vi "AI_Joystick_Manual.vi"() -> ()   [LabVIEW 2016]
uses:
  <vilib>/myRIO/Instrument Drivers/Onboard IO/AI/typedefs/AI Reference.ctl
  <vilib>/myRIO/Common/Instrument Driver Framework/Utilities/typedefs/myRIO Generic Hardware Reference.ctl
  <vilib>/myRIO/Common/Instrument Driver Framework/Utilities/typedefs/Hardware Version Enum.ctl
  <vilib>/myRIO/Common/Instrument Driver Framework/Utilities/typedefs/myRIO v1.0 Reference.ctl
  <vilib>/myRIO/Common/Instrument Driver Framework/Utilities/typedefs/Generic FPGA Reference.ctl
  <vilib>/myRIO/Common/Instrument Driver Framework/myRIO v1.0/AI/typedefs/AI Channels List.ctl
  <vilib>/myRIO/Common/Instrument Driver Framework/myRIO v1.0/AI/typedefs/AI Channels Enum.ctl
  <vilib>/myRIO/Common/Instrument Driver Framework/Utilities/typedefs/Analog Scaling Constants List.ctl
  <vilib>/myRIO/Common/Instrument Driver Framework/Utilities/typedefs/Analog Scaling Constants.ctl
  <vilib>/userdefined/High Color/nirio_resource_hc.ctl
  <vilib>/myRIO/Common/Instrument Driver Framework/Utilities/vis/Is FPGA Ref Available.vi
  <vilib>/myRIO/Common/Instrument Driver Framework/myRIO v1.0/AI/vis/myRIO v1.1 Open AI.vi
  <vilib>/myRIO/Instrument Drivers/Onboard IO/AI/vis/Read.vi
  <vilib>/myRIO/Common/Instrument Driver Framework/Utilities/vis/Validate Channels.vi
  <vilib>/myRIO/Common/Instrument Driver Framework/myRIO v1.0/AI/vis/myRIO v1.0 Reserve AI.vi
  <vilib>/myRIO/Common/Instrument Driver Framework/myRIO v1.0/AI/vis/myRIO v1.0 Build MUX Configuration AI.vi
  <vilib>/myRIO/Common/Instrument Driver Framework/myRIO v1.0/Resource Manager/vis/myRIO v1.0 Reserve Channel List.vi
  <vilib>/myRIO/Common/Instrument Driver Framework/myRIO v1.0/Resource Manager/vis/myRIO v1.0 Reserve Channel.vi
  <vilib>/myRIO/Common/Instrument Driver Framework/myRIO v1.0/Resource Manager/vis/myRIO v1.0 Unreserve Channel.vi
  <vilib>/myRIO/Common/Instrument Driver Framework/myRIO v1.0/Resource Manager/vis/myRIO v1.0 Build Mutex Name.vi
  <vilib>/Utility/VariantDataType/GetNumericInfo.vi
  <vilib>/Utility/error.llb/Error Cluster From Error Code.vi
  <vilib>/myRIO/Common/Instrument Driver Framework/myRIO v1.0/myRIO v1.1 Open.vi
  <vilib>/myRIO/Common/Instrument Driver Framework/myRIO v1.0/AI/vis/myRIO v1.0 Get Scaling Constants AI.vi
  <vilib>/myRIO/Common/Instrument Driver Framework/Utilities/vis/IO Manager.vi
  <vilib>/myRIO/Common/Instrument Driver Framework/Utilities/vis/Configuration Manager.vi
  <vilib>/myRIO/Common/Instrument Driver Framework/myRIO v1.0/myRIO v1.0 Close.vi
  <vilib>/myRIO/Common/Instrument Driver Framework/myRIO v1.0/AI/vis/myRIO v1.0 Read AI.vi
  <vilib>/myRIO/Express VI/Onboard IO/AI/AI Express VI.xnode
  <vilib>/myRIO/Instrument Drivers/Onboard IO/AI/vis/myRIO AI Open.xnode
  <vilib>/myRIO/Instrument Drivers/Onboard IO/AI/AI.lvlib
panel:
  in  "X":dbl=2.0
  in  "y":dbl=2.0
  out "Right Speed":dbl format="%#.1f"
  in  "stop":bool
  out "Reset Encoder":bool
  out "Left Speed":dbl format="%#.1f"
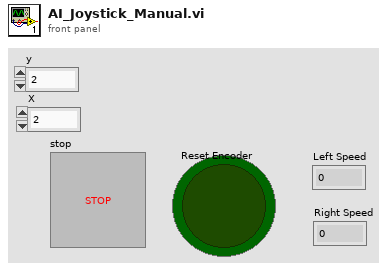
[diagram p1: front panel]
types:
  T1 = typedef "AI.lvlib/AI Reference.ctl" = cluster{"myRIO Reference":T2, "AI Channels List":T6, "AI Scaling Constants List":T8}
  T2 = typedef "myRIO Generic Hardware Reference.ctl" = cluster{"myRIO Model":T3, "myRIO Hardware Reference":T4}
  T3 = typedef "Hardware Version Enum.ctl" = enum16{"Unknown", "myRIO-1900", "myRIO-1950", "roboRIO", "NI ELVIS RIO CM"}
  T4 = typedef "myRIO v1.0 Reference.ctl" = cluster{"Generic FPGA Reference":T5, "Allow multiple opens":bool}
  T5 = typedef "Generic FPGA Reference.ctl" = refnum<k20>
  T6 = typedef "AI Channels List.ctl" = T7[]
  T7 = typedef "AI Channels Enum.ctl" = enum16{"Not Connected", "AudioIn/Left", "AudioIn/Right", "C/AI0", "C/AI1", "A/AI0", "A/AI1", "A/AI2", "A/AI3", "B/AI0", "B/AI1", "B/AI2", "B/AI3", "AI/AI0", "AI/AI1", "AI/AI2", "AI/AI3"}
  T8 = typedef "Analog Scaling Constants List.ctl" = T9[]
  T9 = typedef "Analog Scaling Constants.ctl" = cluster{"LSB Weight (Volts)":dbl, "Offset (Volts)":dbl, "Signed?":bool}
  T10 = typedef "nirio_resource_hc.ctl" = tag
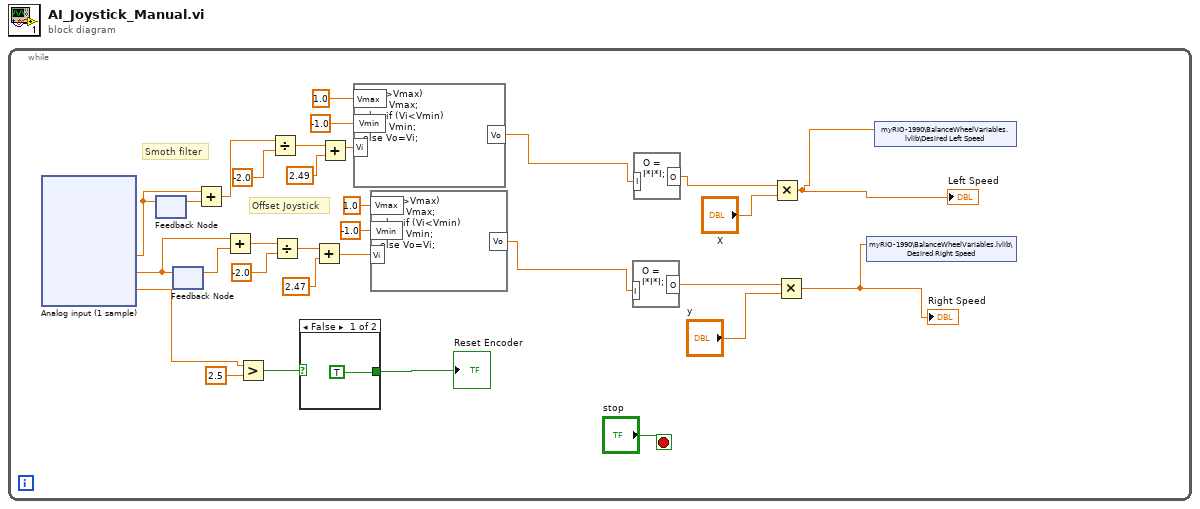
[diagram p0: block diagram]
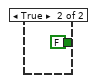
[diagram p2: hidden frame]
diagram:
  n1 = while {
    stop <- "stop" stop-if-true
    # "Offset Joystick"
    # "Smoth filter"
    n2 = xnode "Analog input (1 sample)"() -> ("B/AI2 (Pin 7)"=w18:dbl, "B/AI1 (Pin 5)"=w20:dbl, "B/AI0 (Pin 3)"=w17:dbl)  [unwired: 1 in, 1 out]
    n3 = feedback #1() -> (w27:dbl)  [unwired: 1 in]
    n4 = feedback-in #1(w18) -> ()
    n5 = feedback #2() -> (w23:dbl)  [unwired: 1 in]
    n6 = feedback-in #2(w20) -> ()
    n7 = Add(x=w18, y=w27) -> (x+y=w26:dbl)
    n8 = Add(x=w20, y=w23) -> (x+y=w22:dbl)
    n9 = Greater?(x=w17, y=2.5) -> (0:w30:bool)
    n10 = Divide(x=w26, y=-2.0) -> (x/y=w24:dbl)
    n11 = Divide(x=w22, y=-2.0) -> (x/y=w19:dbl)
    n12 = case shown="False" w30 {
      tunnel: [TRUE ("Boolean 2") FALSE ("Boolean 2")] -> w15
      frame False {
      }
      frame True {
      }
    }
    "Reset Encoder" <- w15
    n13 = Add(x=w19, y=2.47) -> (x+y=w11:dbl)
    n14 = Add(x=w24, y=2.49) -> (x+y=w14:dbl)
    n15 = formula code="if (Vi>Vmax)\nVo = Vmax;\nelse if (Vi<Vmin)\nVo = Vmin;\nelse Vo=Vi;"("Vi"=w14, "Vmin"=-1.0 ("input variable"), "Vmax"=1.0 ("input variable")) -> ("Vo"=w6:dbl)
    n16 = formula code="if (Vi>Vmax)\nVo = Vmax;\nelse if (Vi<Vmin)\nVo = Vmin;\nelse Vo=Vi;"("Vi"=w11, "Vmin"=-1.0 ("input variable"), "Vmax"=1.0 ("input variable")) -> ("Vo"=w4:dbl)
    n17 = formula code="O = I*I*I;"("I"=w4) -> ("O"=w3:dbl)
    n18 = formula code="O = I*I*I;"("I"=w6) -> ("O"=w5:dbl)
    n19 = Multiply(x=w5, y="X") -> (x*y=w2:dbl)
    "Left Speed" <- w2
    n20 = Multiply(x=w3, y="y") -> (x*y=w1:dbl)
    "Right Speed" <- w1
    n21 = shared-variable "myRIO-1990\\BalanceWheelVariables.lvlib\\Desired Right Speed"(w1) -> ()  [unwired: 1 in, 1 out]
    n22 = shared-variable "myRIO-1990\\BalanceWheelVariables.lvlib\\Desired Left Speed"(w2) -> ()  [unwired: 1 in, 1 out]
  }
